vi "Periodic Tasks.vi"(8 "error in":errorcluster) -> ()   [LabVIEW 2014]
doc: "This VI runs in parallel to other tasks. It can contain as many user-defined periodic loops as you need. These can carry out PID or other sorts of timed response."
uses:
  <vilib>/Rock Robotics/WPI/SafetyOutput/WPI_SafetyOutputConfigMenu.ctl
  <vilib>/Rock Robotics/WPI/RobotDrive/WPI_RobotDriveGetSetRefNum.vi
  <vilib>/Rock Robotics/WPI/Joystick/WPI_JoystickGetSetRefNum.vi
  Global 2.vi
  <vilib>/Rock Robotics/WPI/Relay/WPI_RelayValue.ctl
  <vilib>/Analysis/NI_AALBase.lvlib
  <vilib>/Analysis/baseanly.llb/Mean (DBL).vi
panel:
  out "Distance (Inches)":dbl
  out "Raw Voltage":dbl
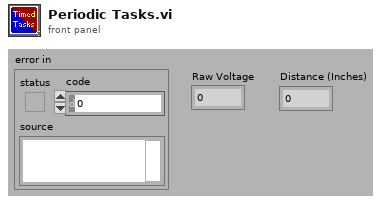
[diagram p1: front panel]
types:
  T1 = typedef "WPI_RobotDriveDevRef.ctl" = cluster{"DevStatus":errorcluster, "Motors[]":T2[], "Square Inputs":bool, "Max Output":dbl}
  T2 = typedef "WPI_MotorControlDeviceRef.ctl" = cluster{"DeviceStatus":errorcluster, "Type":T3, "PWM":cluster{"Controller":T4, "PWM Channel":T5, "DeadBand":T6}, "CAN":cluster{"Device Number":u8, "Control Mode":T7, "Semaphore":T8, "Max Vout":dbl, "TalonSRX Control Mode":T9}, "Invert":bool, "TransformRef":T10, "InvTransformRef":T10}
  T3 = typedef "WPI_MotorControlType.ctl" = enum16{"PWM", "CAN", "CANTalonSRX"}
  T4 = typedef "FPGA_TypedefDigitalModule.ctl" = enum16{"Controller 1"}
  T5 = typedef "FPGA_DIOPWMChannel.ctl" = enum8{"PWM 0", "PWM 1", "PWM 2", "PWM 3", "PWM 4", "PWM 5", "PWM 6", "PWM 7", "PWM 8", "PWM 9", "PWM MXP 0", "PWM MXP 1", "PWM MXP 2", "PWM MXP 3", "PWM MXP 4", "PWM MXP 5", "PWM MXP 6", "PWM MXP 7", "PWM MXP 8", "PWM MXP 9", "Invalid"}
  T6 = typedef "WPI_PWMDeadband.ctl" = cluster{"Name":string, "maxPositivePwm":i32, "minPositivePwm":i32, "centerPwm":i32, "maxNegativePwm":i32, "minNegativePwm":i32, "angularRange":u16}
  T7 = typedef "WPI_CANJaguar_ControlMode.ctl" = enum8{"Percent VBus", "Current", "Speed", "Position", "Voltage"}
  T8 = typedef "Semaphore RefNum" = refnum<k1>
  T9 = typedef "WPI_CANTalonSRX_APIControlMode.ctl" = enum8{"Percent VBus", "Speed", "Position", "Slave", "Unchanged / Invalid"}
  T10 = typedef "WPI_PWMTransform_ConPane.ctl" = refnum<vi>
  T11 = typedef "WPI_JoystickDevRef.ctl" = cluster{"Device":T12}
  T12 = typedef "WPI_JoystickDeviceEnum.ctl" = enum16{"USB 0", "USB 1", "USB 2", "USB 3", "USB 4", "USB 5"}
  T13 = cluster{"JoystickDevRef":T11, "RobotDriveDevRef":T1}
  T14 = typedef "WPI_RelayValue.ctl" = enum16{"Off", "On", "Forward", "Reverse"}
  T15 = typedef "WPI_RelayDevRef.ctl" = cluster{"DevStatus":errorcluster, "Relay Channel":T16, "Controller":T4, "Relay Direction":T17}
  T16 = typedef "FPGA_DIORelayChannel.ctl" = enum8{"Relay 0", "Relay 1", "Relay 2", "Relay 3", "Invalid"}
  T17 = typedef "WPI_RelayDirection.ctl" = enum16{"Both directions", "Forward only", "Reverse only"}
  T18 = typedef "WPI_SafetyOutputConfigMenu.ctl" = enum16{"Enable", "Disable"}
  T19 = typedef "WPI_ServoDeviceRef.ctl" = cluster{"DeviceStatus":errorcluster, "Controller":T4, "PWM Channel":T5, "DeadBand":T6}
  T20 = typedef "WPI_AnalogChannelDevRef.ctl" = cluster{"DevStatus":errorcluster, "Controller":T21, "Analog Channel":T22}
  T21 = typedef "FPGA_TypedefAnalogModule.ctl" = enum16{"Controller 1"}
  T22 = typedef "FPGA_AIChannel.ctl" = enum8{"AI 0", "AI 1", "AI 2", "AI 3", "AI MXP 0", "AI MXP 1", "AI MXP 2", "AI MXP 3", "Invalid"}
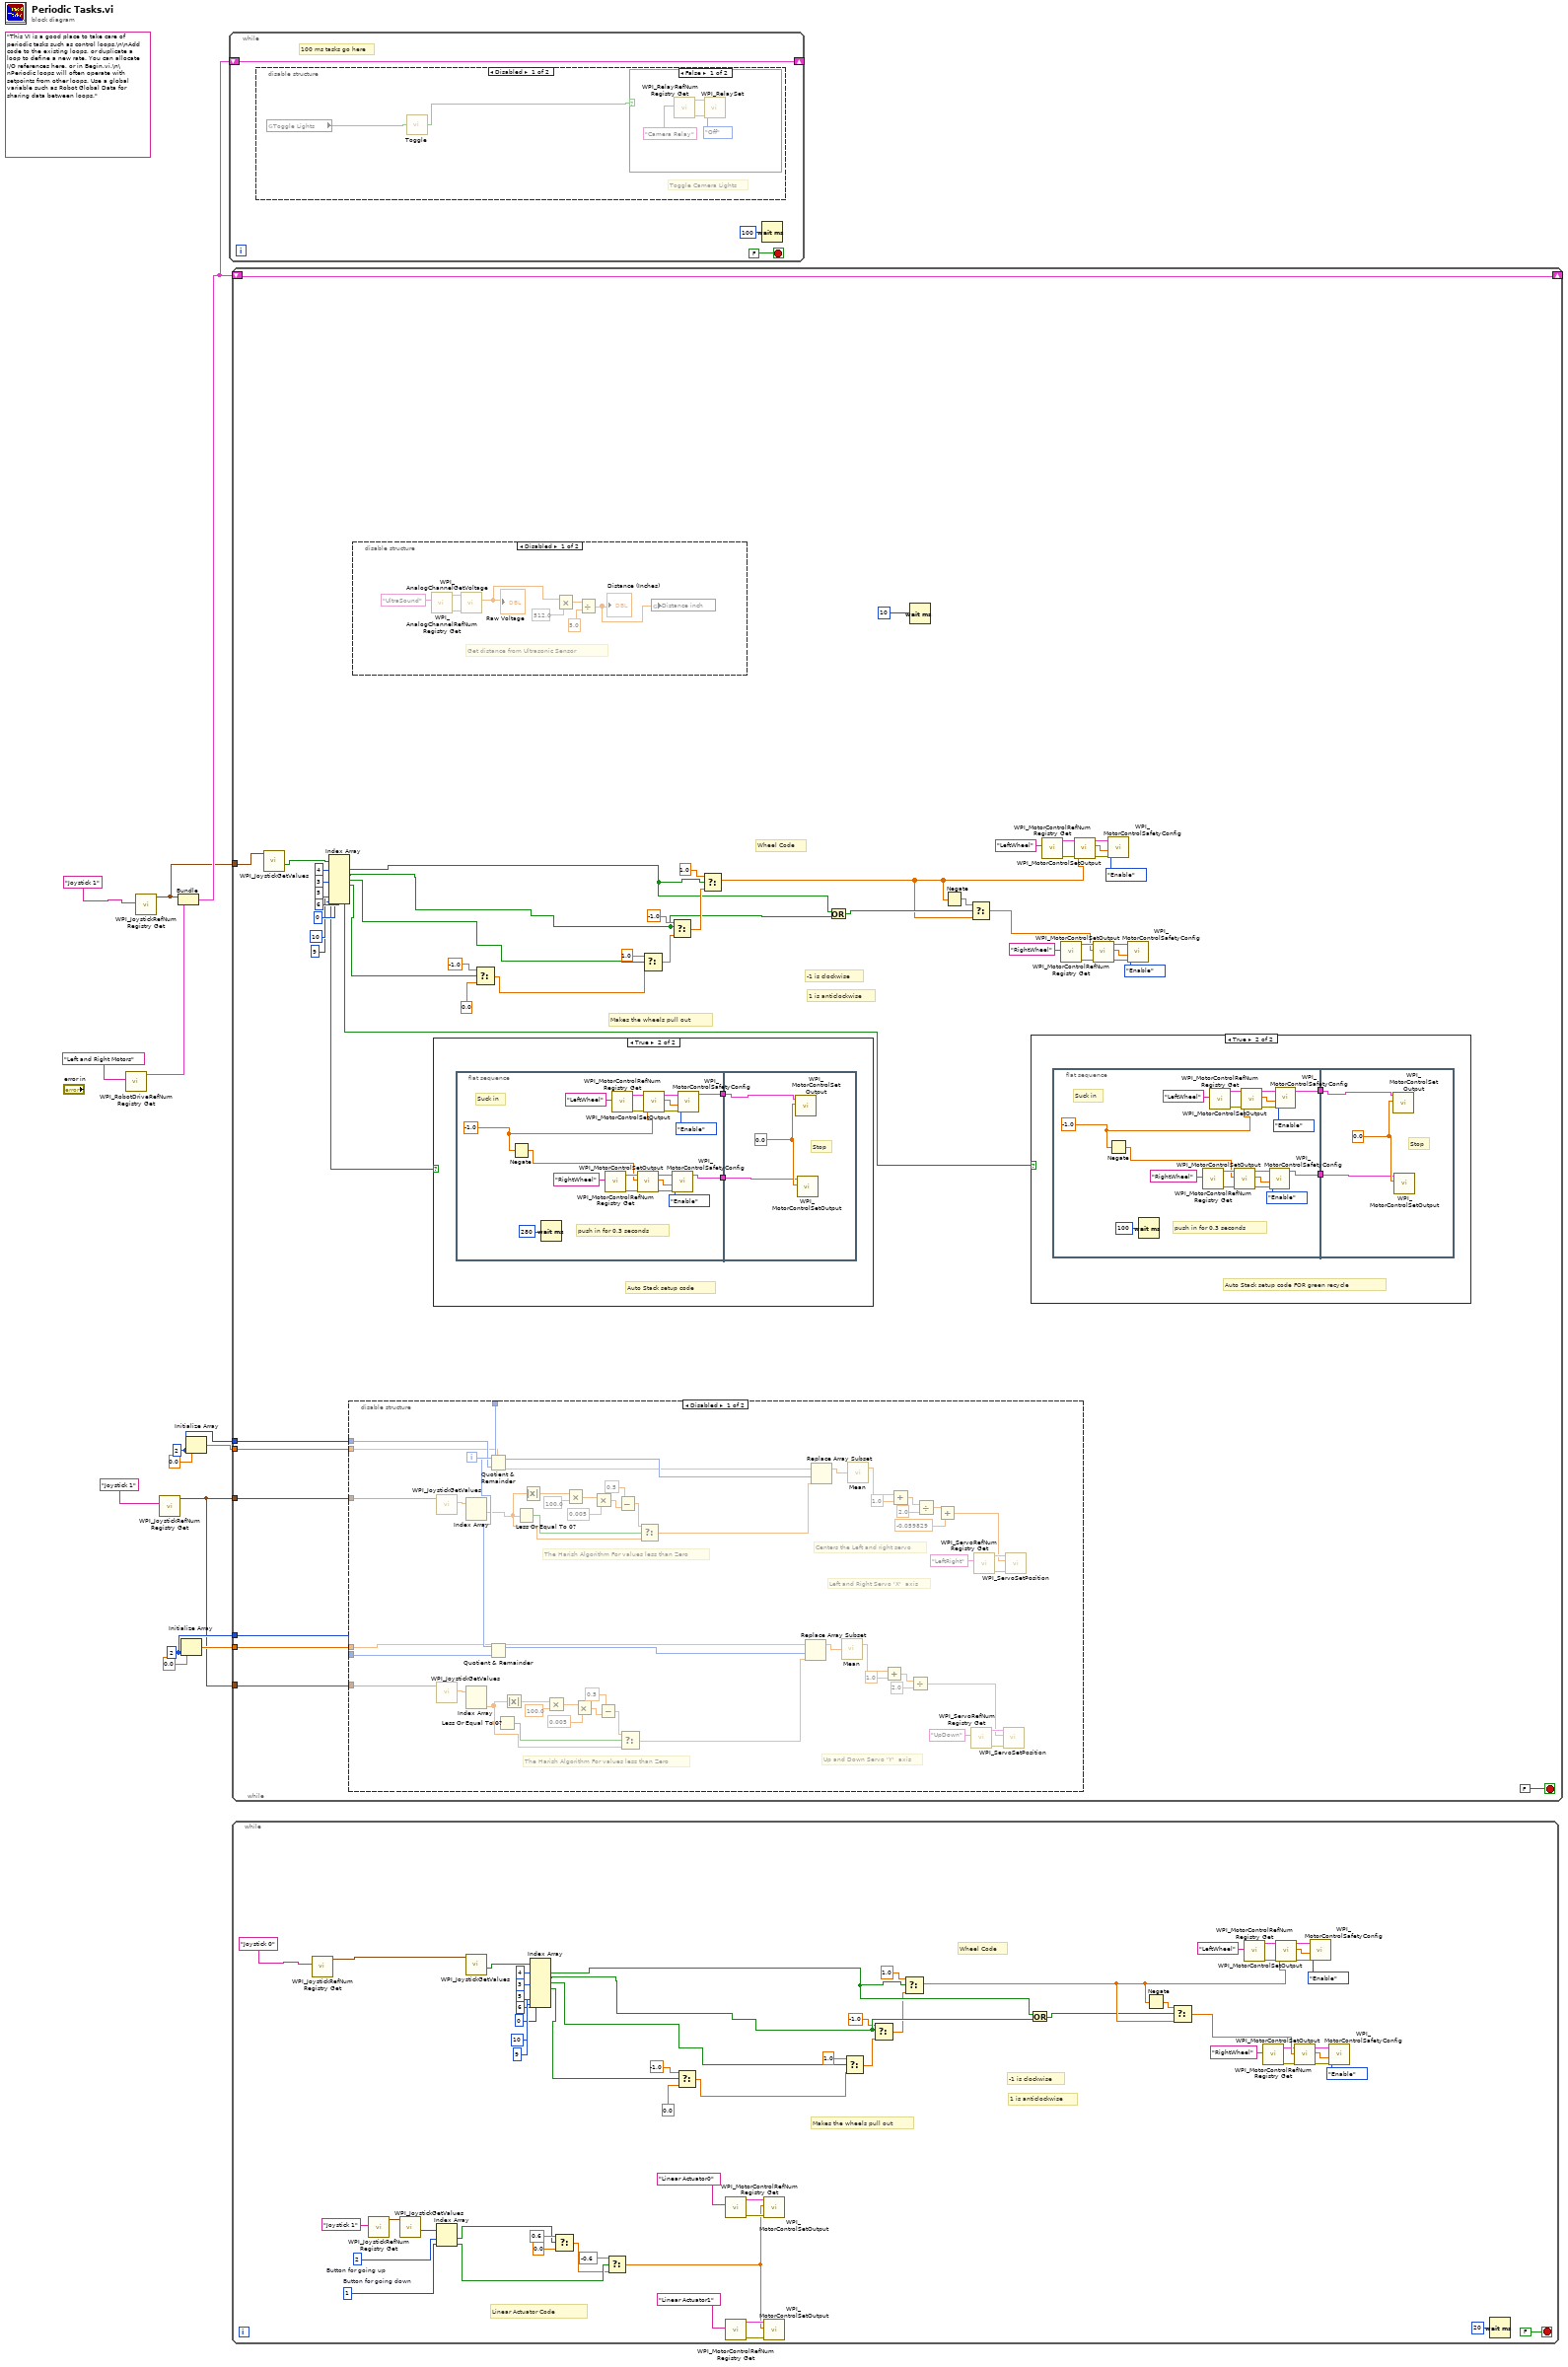
[diagram p0: block diagram]
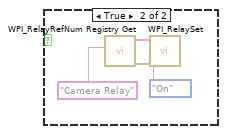
[diagram p6: hidden frame]
diagram:
  w4 = 2 ("index")
  w7 = 2 ("index")
  (unwired) "This VI is a good place to take care of periodic tasks such as control loops.\n\nAdd code to the existing loops, or duplicate a loop to define a new rate. You can allocate I/O references here, or in Begin.vi.\n\nPeriodic loops will often operate with setpoints from other loops. Use a global variable such as Robot Global Data for sharing data between loops."
  n1 = call <vilib>:"WPI_RobotDriveRefNum Registry Get.vi"("refnum name"="Left and Right Motors") -> ("RobotDriveDevRef"=w12:T1)  [unwired: 1 in, 9 out]
  n2 = call <vilib>:"WPI_JoystickRefNum Registry Get.vi"("refnum name"="Joystick 1") -> ("JoystickDevRef"=w10:T11)  [unwired: 1 in, 9 out]
  n3 = call <vilib>:"WPI_JoystickRefNum Registry Get.vi"("refnum name"="Joystick 1") -> ("JoystickDevRef"=w2:T11)  [unwired: 1 in, 9 out]
  n4 = Bundle("JoystickDevRef"=w10, "RobotDriveDevRef"=w12) -> (w11:T13)  [unwired: 1 out]
  n5 = Initialize Array(0.0 ("element"), w4) -> (w3:dbl[])
  n6 = Initialize Array(0.0 ("element"), w7) -> (w5:dbl[])
  n7 = while {
    shift-right: [w14] -> _
    shift-left: w11 -> [w14]
    stop <- FALSE stop-if-true
    # "100 ms tasks go here"
    n8 = disable-structure shown="Disabled" {
      frame Disabled {
        # "Toggle Camera Lights"
        n9 = global read "Global 2.vi" "Toggle Lights"() -> (w18:bool)
        n10 = call "Toggle.vi"("Input"=w18) -> ("Output"=w17:bool)
        n11 = case shown="False" w17 {
          frame False {
            n12 = call <vilib>:"WPI_RelayRefNum Registry Get.vi"("refnum name"="Camera Relay") -> ("error out"=w21:errorcluster, "RelayDevRef"=w20:T15)  [unwired: 9 in]
            n13 = call <vilib>:"WPI_RelaySet.vi"("error in (no error)"=w21, "RelayValue"=WPI_RelayValue."Off", "RelayDevRef"=w20) -> ()  [unwired: 7 in, 2 out]
          }
          frame True {
            n14 = call <vilib>:"WPI_RelayRefNum Registry Get.vi"("refnum name"="Camera Relay") -> ("error out"=w25:errorcluster, "RelayDevRef"=w24:T15)  [unwired: 9 in]
            n15 = call <vilib>:"WPI_RelaySet.vi"("error in (no error)"=w25, "RelayValue"=WPI_RelayValue."On", "RelayDevRef"=w24) -> ()  [unwired: 7 in, 2 out]
          }
        }
      }
      frame Enabled {
      }
    }
    n16 = Wait (ms)(milliseconds to wait=u32 100) -> ()  [unwired: 1 out]
  }
  n17 = while {
    shift-right: [w75] -> _
    shift-left: w11 -> [w75]
    tunnel: w10 -> [w36]
    tunnel: w2 -> [w35]
    tunnel: w7 -> [w34]
    tunnel: w5 -> [w33]
    tunnel: w4 -> [w32]
    tunnel: w3 -> [w30]
    tunnel: w2 -> [w29]
    i -> [w31]
    stop <- FALSE stop-if-true
    # "Wheel Code"
    # "1 is anticlockwise"
    # "-1 is clockwise"
    # "Makes the wheels pull out"
    n18 = call <vilib>:"WPI_JoystickGetValues.vi"("JoystickDevRef"=w36) -> ("Buttons"=w40:bool[])  [unwired: 6 in, 4 out]
    n19 = Index Array(array=w40, index #1=4 ("index"), index #2=3 ("index"), index #3=5 ("index"), index #4=6 ("index"), index #5=0 ("index"), index #6=10 ("index"), index #7=9 ("index")) -> (element #1=w41:bool, element #2=w42:bool, element #3=w43:bool, element #4=w47:bool, element #5=w38:bool, element #7=w27:bool)  [unwired: 1 out]
    n20 = disable-structure shown="Disabled" {
      disable-tunnel: w35 -> [w128 _]
      disable-tunnel: w34 -> [w117 _]
      disable-tunnel: w33 -> [w105 _]
      disable-tunnel: w32 -> [w104 _]
      disable-tunnel: w31 -> [w103 _]
      disable-tunnel: w30 -> [w102 _]
      disable-tunnel: w29 -> [w101 _]
      frame Disabled {
        # "Centers the Left and right servo"
        # "The Harish Algorithm For values less than Zero"
        # "The Harish Algorithm For values less than Zero"
        # "Up and Down Servo 'Y'  axis"
        # "Left and Right Servo 'X'  axis"
        n21 = call <vilib>:"WPI_JoystickGetValues.vi"("JoystickDevRef"=w128) -> ("Axes"=w124:dbl[])  [unwired: 6 in, 4 out]
        n22 = call <vilib>:"WPI_JoystickGetValues.vi"("JoystickDevRef"=w101) -> ("Axes"=w113:dbl[])  [unwired: 6 in, 4 out]
        n23 = Index Array(array=w124) -> (element #1=w79:dbl)  [unwired: 2 in, 1 out]
        n24 = Index Array(array=w113) -> (element #2=w96:dbl)  [unwired: 2 in, 1 out]
        n25 = Quotient & Remainder(x=w103, y=w117) -> (x-y*floor(x/y)=w123:i32)  [unwired: 1 out]
        n26 = Quotient & Remainder(x=w103, y=w104) -> (x-y*floor(x/y)=w112:i32)  [unwired: 1 out]
        n27 = Less Or Equal To 0?(x=w96) -> (x <= 0?=w97:bool)
        n28 = Absolute Value(x=w96) -> (abs(x)=w94:dbl)
        n29 = Less Or Equal To 0?(x=w79) -> (x <= 0?=w87:bool)
        n30 = Absolute Value(x=w79) -> (abs(x)=w85:dbl)
        n31 = Multiply(x=w94, y=100.0) -> (x*y=w93:dbl)
        n32 = Multiply(x=w85, y=100.0) -> (x*y=w84:dbl)
        n33 = Multiply(x=w93, y=0.005) -> (x*y=w88:dbl)
        n34 = Multiply(x=w84, y=0.005) -> (x*y=w80:dbl)
        n35 = Subtract(x=0.5 ("y"), y=w88) -> (x-y=w91:dbl)
        n36 = Subtract(x=0.5 ("y"), y=w80) -> (x-y=w82:dbl)
        n37 = Select(t=w91, s=w97, f=w96) -> (s? t:f=w90:dbl)
        n38 = Select(t=w82, s=w87, f=w79) -> (s? t:f=w78:dbl)
        n39 = Replace Array Subset(array=w102, new element=w90, index=w112) -> (w111:dbl[])
        n40 = Replace Array Subset(array=w105, new element=w78, index=w123) -> (w122:dbl[])
        n41 = call-poly <vilib>:"Mean.vi"("X"=w111) -> ("mean"=w110:dbl)  [unwired: 1 out]
        n42 = call-poly <vilib>:"Mean.vi"("X"=w122) -> ("mean"=w121:dbl)  [unwired: 1 out]
        n43 = Add(x=w110, y=1.0) -> (x+y=w108:dbl)
        n44 = Add(x=w121, y=1.0) -> (x+y=w119:dbl)
        n45 = Divide(x=w108, y=2.0) -> (x/y=w106:dbl)
        n46 = Divide(x=w119, y=2.0) -> (x/y=w100:dbl)
        n47 = Add(x=w100, y=-0.059829) -> (x+y=w98:dbl)
        n48 = call <vilib>:"WPI_ServoRefNum Registry Get.vi"("refnum name"="UpDown") -> ("error out"=w115:errorcluster, "ServoDeviceRef"=w114:T19)  [unwired: 9 in]
        n49 = call <vilib>:"WPI_ServoRefNum Registry Get.vi"("refnum name"="LeftRight") -> ("error out"=w126:errorcluster, "ServoDeviceRef"=w125:T19)  [unwired: 9 in]
        n50 = call <vilib>:"WPI_ServoSetPosition.vi"("error in (no error)"=w115, "Position"=w106, "ServoDeviceRef"=w114) -> ()  [unwired: 7 in, 2 out]
        n51 = call <vilib>:"WPI_ServoSetPosition.vi"("error in (no error)"=w126, "Position"=w98, "ServoDeviceRef"=w125) -> ()  [unwired: 7 in, 2 out]
      }
      frame Enabled {
      }
    }
    n52 = disable-structure shown="Disabled" {
      frame Disabled {
        # "Get distance from Ultrasonic Sensor"
        n53 = call <vilib>:"WPI_AnalogChannelRefNum Registry Get.vi"("refnum name"="UltraSound") -> ("error out"=w159:errorcluster, "AIDeviceRef"=w158:T20)  [unwired: 9 in]
        n54 = call <vilib>:"WPI_AnalogChannelGetVoltage.vi"("error in (no error)"=w159, "AIDeviceRef"=w158) -> ("Voltage"=w157:dbl)  [unwired: 7 in, 2 out]
        "Raw Voltage" <- w157
        n55 = Multiply(x=w157, y=512.0) -> (x*y=w155:dbl)
        n56 = Divide(x=w155, y=5.0) -> (x/y=w153:dbl)
        "Distance (Inches)" <- w153
        n57 = global write "Global 2.vi" "Distance inch"(w153) -> ()
      }
      frame Enabled {
      }
    }
    n58 = case shown="True" w38 {
      frame False {
      }
      frame True {
        # "Auto Stack setup code"
        n59 = flat-sequence {
          tunnel: [w164] -> w162
          tunnel: [w163] -> w161
          tunnel: w162 -> [w182]
          tunnel: w161 -> [w183]
          frame #0 {
            w166 = -1.0
            # "Suck in"
            # "push in for 0.3 seconds"
            n60 = Negate(x=w166) -> (-x=w167:dbl)
            n61 = Wait (ms)(milliseconds to wait=u32 280) -> ()  [unwired: 1 out]
            n62 = call <vilib>:"WPI_MotorControlRefNum Registry Get.vi"("refnum name"="RightWheel") -> ("error out"=w179:errorcluster, "MotorControlDevRef"=w178:T2)  [unwired: 9 in]
            n63 = call <vilib>:"WPI_MotorControlRefNum Registry Get.vi"("refnum name"="LeftWheel") -> ("error out"=w181:errorcluster, "MotorControlDevRef"=w180:T2)  [unwired: 9 in]
            n64 = call <vilib>:"WPI_MotorControlSetOutput.vi"("error in (no error)"=w179, "Output"=w167, "MotorControlDevRef"=w178) -> ("error out"=w172:errorcluster, "Motor Output"=w171:dbl, "MotorControlDevRef"=w170:T2)  [unwired: 6 in]
            n65 = call <vilib>:"WPI_MotorControlSetOutput.vi"("error in (no error)"=w181, "Output"=w166, "MotorControlDevRef"=w180) -> ("error out"=w175:errorcluster, "Motor Output"=w174:dbl, "MotorControlDevRef"=w173:T2)  [unwired: 6 in]
            n66 = call <vilib>:"WPI_MotorControlSafetyConfig.vi"("error in (no error)"=w172, "timeout (s)"=w171, "mode"=WPI_SafetyOutputConfigMenu."Enable", "MotorControlDevRef"=w170) -> ("MotorControlDevRef"=w164:T2)  [unwired: 6 in, 1 out]
            n67 = call <vilib>:"WPI_MotorControlSafetyConfig.vi"("error in (no error)"=w175, "timeout (s)"=w174, "mode"=WPI_SafetyOutputConfigMenu."Enable", "MotorControlDevRef"=w173) -> ("MotorControlDevRef"=w163:T2)  [unwired: 6 in, 1 out]
          }
          frame #1 {
            w184 = 0.0
            # "Stop"
            n68 = call <vilib>:"WPI_MotorControlSetOutput.vi"("Output"=w184, "MotorControlDevRef"=w183) -> ()  [unwired: 7 in, 3 out]
            n69 = call <vilib>:"WPI_MotorControlSetOutput.vi"("Output"=w184, "MotorControlDevRef"=w182) -> ()  [unwired: 7 in, 3 out]
          }
        }
      }
    }
    n70 = Select(t=-1.0, s=w47, f=0.0) -> (s? t:f=w44:dbl)
    n71 = Select(t=1.0, s=w43, f=w44) -> (s? t:f=w57:dbl)
    n72 = Select(t=-1.0, s=w42, f=w57) -> (s? t:f=w58:dbl)
    n73 = Select(t=1.0, s=w41, f=w58) -> (s? t:f=w52:dbl)
    n74 = Or(x=w41, y=w42) -> (x .or. y?=w54:bool)
    n75 = Wait (ms)(milliseconds to wait=u32 10) -> ()  [unwired: 1 out]
    n76 = Negate(x=w52) -> (-x=w53:dbl)
    n77 = Select(t=w53, s=w54, f=w52) -> (s? t:f=w55:dbl)
    n78 = case shown="True" w27 {
      frame False {
      }
      frame True {
        # "Auto Stack setup code FOR green recycle"
        n79 = flat-sequence {
          tunnel: [w132] -> w130
          tunnel: [w131] -> w129
          tunnel: w130 -> [w150]
          tunnel: w129 -> [w151]
          frame #0 {
            w134 = -1.0
            # "Suck in"
            # "push in for 0.3 seconds"
            n80 = Negate(x=w134) -> (-x=w135:dbl)
            n81 = Wait (ms)(milliseconds to wait=u32 100) -> ()  [unwired: 1 out]
            n82 = call <vilib>:"WPI_MotorControlRefNum Registry Get.vi"("refnum name"="RightWheel") -> ("error out"=w147:errorcluster, "MotorControlDevRef"=w146:T2)  [unwired: 9 in]
            n83 = call <vilib>:"WPI_MotorControlRefNum Registry Get.vi"("refnum name"="LeftWheel") -> ("error out"=w149:errorcluster, "MotorControlDevRef"=w148:T2)  [unwired: 9 in]
            n84 = call <vilib>:"WPI_MotorControlSetOutput.vi"("error in (no error)"=w147, "Output"=w135, "MotorControlDevRef"=w146) -> ("error out"=w140:errorcluster, "Motor Output"=w139:dbl, "MotorControlDevRef"=w138:T2)  [unwired: 6 in]
            n85 = call <vilib>:"WPI_MotorControlSetOutput.vi"("error in (no error)"=w149, "Output"=w134, "MotorControlDevRef"=w148) -> ("error out"=w143:errorcluster, "Motor Output"=w142:dbl, "MotorControlDevRef"=w141:T2)  [unwired: 6 in]
            n86 = call <vilib>:"WPI_MotorControlSafetyConfig.vi"("error in (no error)"=w140, "timeout (s)"=w139, "mode"=WPI_SafetyOutputConfigMenu."Enable", "MotorControlDevRef"=w138) -> ("MotorControlDevRef"=w132:T2)  [unwired: 6 in, 1 out]
            n87 = call <vilib>:"WPI_MotorControlSafetyConfig.vi"("error in (no error)"=w143, "timeout (s)"=w142, "mode"=WPI_SafetyOutputConfigMenu."Enable", "MotorControlDevRef"=w141) -> ("MotorControlDevRef"=w131:T2)  [unwired: 6 in, 1 out]
          }
          frame #1 {
            w152 = 0.0
            # "Stop"
            n88 = call <vilib>:"WPI_MotorControlSetOutput.vi"("Output"=w152, "MotorControlDevRef"=w151) -> ()  [unwired: 7 in, 3 out]
            n89 = call <vilib>:"WPI_MotorControlSetOutput.vi"("Output"=w152, "MotorControlDevRef"=w150) -> ()  [unwired: 7 in, 3 out]
          }
        }
      }
    }
    n90 = call <vilib>:"WPI_MotorControlRefNum Registry Get.vi"("refnum name"="LeftWheel") -> ("error out"=w73:errorcluster, "MotorControlDevRef"=w72:T2)  [unwired: 9 in]
    n91 = call <vilib>:"WPI_MotorControlRefNum Registry Get.vi"("refnum name"="RightWheel") -> ("error out"=w71:errorcluster, "MotorControlDevRef"=w70:T2)  [unwired: 9 in]
    n92 = call <vilib>:"WPI_MotorControlSetOutput.vi"("error in (no error)"=w73, "Output"=w52, "MotorControlDevRef"=w72) -> ("error out"=w67:errorcluster, "Motor Output"=w66:dbl, "MotorControlDevRef"=w65:T2)  [unwired: 6 in]
    n93 = call <vilib>:"WPI_MotorControlSetOutput.vi"("error in (no error)"=w71, "Output"=w55, "MotorControlDevRef"=w70) -> ("error out"=w64:errorcluster, "Motor Output"=w63:dbl, "MotorControlDevRef"=w62:T2)  [unwired: 6 in]
    n94 = call <vilib>:"WPI_MotorControlSafetyConfig.vi"("error in (no error)"=w67, "timeout (s)"=w66, "mode"=WPI_SafetyOutputConfigMenu."Enable", "MotorControlDevRef"=w65) -> ()  [unwired: 6 in, 2 out]
    n95 = call <vilib>:"WPI_MotorControlSafetyConfig.vi"("error in (no error)"=w64, "timeout (s)"=w63, "mode"=WPI_SafetyOutputConfigMenu."Enable", "MotorControlDevRef"=w62) -> ()  [unwired: 6 in, 2 out]
  }
  n96 = while {
    stop <- FALSE stop-if-true
    w202 = 1  # Button for going down
    w203 = 2  # Button for going up
    # "Linear Actuator Code"
    # "Wheel Code"
    # "1 is anticlockwise"
    # "-1 is clockwise"
    # "Makes the wheels pull out"
    n97 = call <vilib>:"WPI_JoystickRefNum Registry Get.vi"("refnum name"="Joystick 0") -> ("JoystickDevRef"=w187:T11)  [unwired: 1 in, 9 out]
    n98 = call <vilib>:"WPI_JoystickRefNum Registry Get.vi"("refnum name"="Joystick 1") -> ("JoystickDevRef"=w205:T11)  [unwired: 9 in, 1 out]
    n99 = call <vilib>:"WPI_JoystickGetValues.vi"("JoystickDevRef"=w205) -> ("Buttons"=w204:bool[])  [unwired: 6 in, 4 out]
    n100 = Index Array(array=w204, index #1=w203, index #2=w202) -> (element #1=w194:bool, element #2=w195:bool)
    n101 = call <vilib>:"WPI_JoystickGetValues.vi"("JoystickDevRef"=w187) -> ("Buttons"=w241:bool[])  [unwired: 6 in, 4 out]
    n102 = Index Array(array=w241, index #1=4 ("index"), index #2=3 ("index"), index #3=5 ("index"), index #4=6 ("index"), index #5=0 ("index"), index #6=10 ("index"), index #7=9 ("index")) -> (element #1=w240:bool, element #2=w239:bool, element #3=w238:bool, element #4=w234:bool)  [unwired: 3 out]
    n103 = Select(t=0.6, s=w194, f=0.0) -> (s? t:f=w193:dbl)
    n104 = Select(t=-0.6, s=w195, f=w193) -> (s? t:f=w189:dbl)
    n105 = Select(t=-1.0, s=w234, f=0.0) -> (s? t:f=w237:dbl)
    n106 = call <vilib>:"WPI_MotorControlRefNum Registry Get.vi"("refnum name"="Linear Actuator0") -> ("error out"=w201:errorcluster, "MotorControlDevRef"=w200:T2)  [unwired: 9 in]
    n107 = call <vilib>:"WPI_MotorControlRefNum Registry Get.vi"("refnum name"="Linear Actuator1") -> ("error out"=w192:errorcluster, "MotorControlDevRef"=w191:T2)  [unwired: 9 in]
    n108 = call <vilib>:"WPI_MotorControlSetOutput.vi"("error in (no error)"=w201, "Output"=w189, "MotorControlDevRef"=w200) -> ()  [unwired: 6 in, 3 out]
    n109 = call <vilib>:"WPI_MotorControlSetOutput.vi"("error in (no error)"=w192, "Output"=w189, "MotorControlDevRef"=w191) -> ()  [unwired: 6 in, 3 out]
    n110 = Select(t=1.0, s=w238, f=w237) -> (s? t:f=w224:dbl)
    n111 = Select(t=-1.0, s=w239, f=w224) -> (s? t:f=w223:dbl)
    n112 = Select(t=1.0, s=w240, f=w223) -> (s? t:f=w229:dbl)
    n113 = Or(x=w240, y=w239) -> (x .or. y?=w227:bool)
    n114 = Negate(x=w229) -> (-x=w228:dbl)
    n115 = Select(t=w228, s=w227, f=w229) -> (s? t:f=w226:dbl)
    n116 = call <vilib>:"WPI_MotorControlRefNum Registry Get.vi"("refnum name"="LeftWheel") -> ("error out"=w208:errorcluster, "MotorControlDevRef"=w209:T2)  [unwired: 9 in]
    n117 = call <vilib>:"WPI_MotorControlRefNum Registry Get.vi"("refnum name"="RightWheel") -> ("error out"=w210:errorcluster, "MotorControlDevRef"=w211:T2)  [unwired: 9 in]
    n118 = call <vilib>:"WPI_MotorControlSetOutput.vi"("error in (no error)"=w208, "Output"=w229, "MotorControlDevRef"=w209) -> ("error out"=w214:errorcluster, "Motor Output"=w215:dbl, "MotorControlDevRef"=w216:T2)  [unwired: 6 in]
    n119 = call <vilib>:"WPI_MotorControlSetOutput.vi"("error in (no error)"=w210, "Output"=w226, "MotorControlDevRef"=w211) -> ("error out"=w217:errorcluster, "Motor Output"=w218:dbl, "MotorControlDevRef"=w219:T2)  [unwired: 6 in]
    n120 = call <vilib>:"WPI_MotorControlSafetyConfig.vi"("error in (no error)"=w214, "timeout (s)"=w215, "mode"=WPI_SafetyOutputConfigMenu."Enable", "MotorControlDevRef"=w216) -> ()  [unwired: 6 in, 2 out]
    n121 = call <vilib>:"WPI_MotorControlSafetyConfig.vi"("error in (no error)"=w217, "timeout (s)"=w218, "mode"=WPI_SafetyOutputConfigMenu."Enable", "MotorControlDevRef"=w219) -> ()  [unwired: 6 in, 2 out]
    n122 = Wait (ms)(milliseconds to wait=u32 20) -> ()  [unwired: 1 out]
  }
